vi "Read_Wrap_Simple.vi"(4 "Numeric in":refnum<class "Var_EXT.lvclass">) -> (1 "Value":T1)   [LabVIEW 2021, in "Var_EXT.lvclass"]
uses:
  Var_EXT.lvclass
  Type.ctl
  Var_EXT.lvclass/Var_EXT.ctl
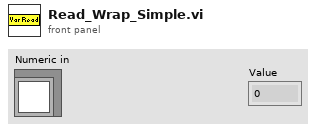
[diagram p1: front panel]
types:
  T1 = typedef "Var_EXT.lvclass/Type.ctl" = dbl
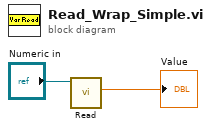
[diagram p0: block diagram]
diagram:
  n1 = call-dynamic "Read.vi"("Numeric in"="Numeric in") -> ("Numeric"=→"Value":T1)  [unwired: 8 in, 2 out]
